vi "DI.vi"() -> ()   [LabVIEW 2025]
uses:
  <vilib>/DAQmx/read.llb/DAQmx Read (Digital 1D Wfm NChan NSamp).vi
  <vilib>/DAQmx/configure/timing.llb/DAQmx Timing (Sample Clock).vi
  <vilib>/DAQmx/miscellaneous.llb/DAQmx Fill In Error Info.vi
  <vilib>/DAQmx/create/channels.llb/DAQmx Create Channel (AI-Voltage-Basic).vi
panel:
  in  "stop":bool
  out "Digital Waveform Graph":digitalwaveform[](graph)
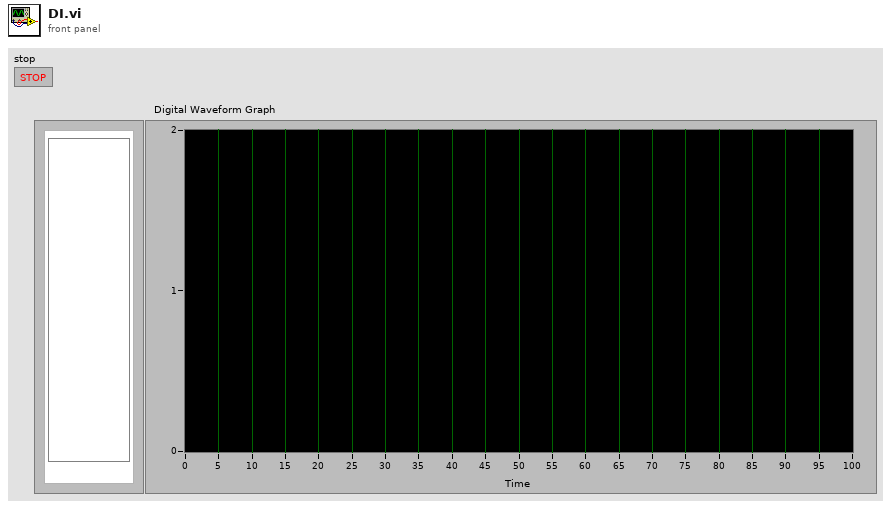
[diagram p1: front panel]
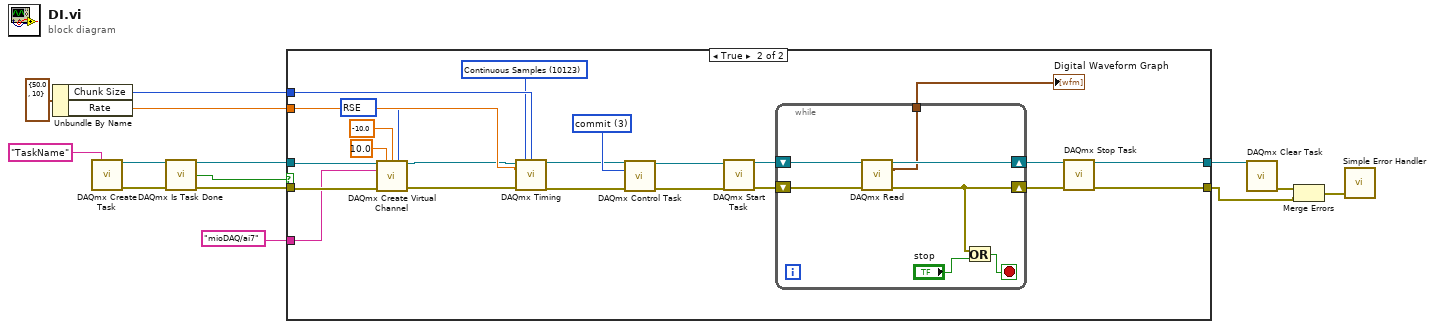
[diagram p0: block diagram]
diagram:
  n1 = Unbundle By Name(cluster{"Rate":dbl, "Chunk Size":i32} {"Rate"=50.0, "Chunk Size"=10} ("input cluster")) -> ("Chunk Size"=w12:i32, "Rate"=w13:dbl)
  n2 = call <vilib>:"DAQmx Create Task.vi"("new task name"="TaskName") -> ("task out"=w2:refnum<k21>, "error out"=w3:errorcluster)  [unwired: 13 in]
  n3 = call <vilib>:"DAQmx Is Task Done.vi"("task/channels in"=w2, "error in"=w3) -> ("task out"=w9:refnum<k21>, "task done?"=w7:bool, "error out"=w8:errorcluster)  [unwired: 11 in]
  n4 = case shown="True" w7 {
    tunnel: w13 -> [_ w36]
    tunnel: w12 -> [_ w35]
    tunnel: [w16 w27] -> w10
    tunnel: w9 -> [w16 w17]
    tunnel: w8 -> [w15 w22]
    tunnel: [w15 w25] -> w5
    tunnel: "mioDAQ/ai7" ("new task name") -> [_ w19]
    frame False {
    }
    frame True {
      w18 = 10083 items=["Default"=-1, "RSE"=10083, "NRSE"=10078, "Differential"=10106, "Pseudodifferential"=12529] ("input terminal configuration")
      w39 = 3 items=["verify"=2, "reserve"=4, "commit"=3, "unreserve"=5, "abort"=6] ("action")
      w34 = 10123 items=["Finite Samples"=10178, "Continuous Samples"=10123, "Hardware Timed Single Point"=12522] ("sample mode")
      n5 = call-poly <vilib>:"DAQmx Create Virtual Channel.vi"("task in"=w17, "maximum value"=10.0, "minimum value"=-10.0, "input terminal configuration"=w18, "physical channels"=w19, "error in"=w22) -> ("task out"=w24:refnum<k21>, "error out"=w23:errorcluster)  [unwired: 8 in]
      n6 = call-poly <vilib>:"DAQmx Timing.vi"("task/channels in"=w24, "sample mode"=w34, "samples per channel"=w35, "rate"=w36, "error in"=w23) -> ("task out"=w37:refnum<k21>, "error out"=w38:errorcluster)  [unwired: 9 in]
      n7 = call <vilib>:"DAQmx Control Task.vi"("task/channels in"=w37, "action"=w39, "error in"=w38) -> ("task out"=w33:refnum<k21>, "error out"=w32:errorcluster)  [unwired: 11 in]
      n8 = call <vilib>:"DAQmx Start Task.vi"("task/channels in"=w33, "error in"=w32) -> ("task out"=w31:refnum<k21>, "error out"=w30:errorcluster)  [unwired: 12 in]
      n9 = while {
        tunnel: [w43] -> w26
        shift-right: [w44] -> w29
        shift-left: w31 -> [w46]
        shift-right: [w40] -> w28
        shift-left: w30 -> [w45]
        stop <- w41 stop-if-true
        n10 = call-poly <vilib>:"DAQmx Read.vi"("task/channels in"=w46, "error in"=w45) -> ("task out"=w44:refnum<k21>, "data"=w43:digitalwaveform[], "error out"=w40:errorcluster)  [unwired: 11 in]
        n11 = Or(x=w40, y="stop") -> (x .or. y?=w41:bool)
      }
      "Digital Waveform Graph" <- w26
      n12 = call <vilib>:"DAQmx Stop Task.vi"("task/channels in"=w29, "error in"=w28) -> ("task out"=w27:refnum<k21>, "error out"=w25:errorcluster)  [unwired: 12 in]
    }
  }
  n13 = call <vilib>:"DAQmx Clear Task.vi"("task in"=w10) -> ("error out"=w6:errorcluster)  [unwired: 14 in]
  n14 = Merge Errors(w6, w5) -> (w4:errorcluster)
  n15 = call <vilib>:"Simple Error Handler.vi"("error in (no error)"=w4) -> ()  [unwired: 4 in, 5 out]
